vi "CD Read Engine.vi"(5 "Inline Status Channels Refs":T2[](array[typedef]) format="%.0x", 7 "Error (in)":errorcluster, 8 "RT Inline Data_Data Description_Channels":T3[](array[typedef]) {"Frame Drescriptors"."RT"."Status Channel Ref" format="%.0x"; "Frame Drescriptors"."RT"."Words Block Data Refs"."Data Reference" format="%.0x"; "Frame Drescriptors"."RT"."Timestamp Channel Data Reference" format="%.0x"; "Frame Drescriptors"."BC"."Status Channel Refs" format="%.0x"; "Frame Drescriptors"."BC"."Words Block Data Refs"."Data Reference" format="%.0x"; "Frame Drescriptors"."BC"."Timestamp Channel Data Reference" format="%.0x"}, 9 "Card Parameters (in)":T12) -> (0 "Error (out)":errorcluster, 3 "Array":T1[](array[typedef]) {"type" format="%04x"; "activity" format="%04x"; "error" format="%04x"; "cwd1" format="%04x"; "cwd2" format="%04x"; "swd1" format="%04x"; "swd2" format="%04x"; "data" format="%04x"})   [LabVIEW 2020, in "Ballard MIL-1553 Engine.lvlib"]
uses:
  Ballard MIL-1553 Engine.lvlib
  Controls/RT Inline Data_Data Description_Channel.ctl
  Controls/RT Inline Frame Descriptor.ctl
  Controls/RT Inline Frame Descriptor_BC.ctl
  <vilib>/NI VeriStand/Custom Device API/Data Reference.ctl
  <vilib>/NI VeriStand/Custom Device API/Block Data Reference.ctl
  <vilib>/NI VeriStand/Custom Device API/Custom Device Item Ref.ctl
  Controls/RT Inline Frame Descriptor_RT.ctl
  Shared/Controls and Global/RT CWD2.ctl
  Shared/Controls and Global/RT CWD1.ctl
  Shared/Controls and Global/RT messageType.ctl
  Controls/Card Parameters.ctl
  Shared/Controls and Global/Initialization Method.ctl
  <instrlib>/BTICardLib/Public/Controls/1553 Record.ctl
  <instrlib>/BTICardLib/BTICardLV.lvlib
  <vilib>/NI VeriStand/Custom Device Tools/Custom Device Utility Library/Custom Device Utility Library.lvlib
  Shared/Ballard 1553 Shared.lvlib
  <vilib>/NI VeriStand/Custom Device API/Custom Device API.lvlib
panel:
  in  "Tab Control":enum32{"Controls & Indicators", "Misc"}(tab)
  out "# of records read":i32
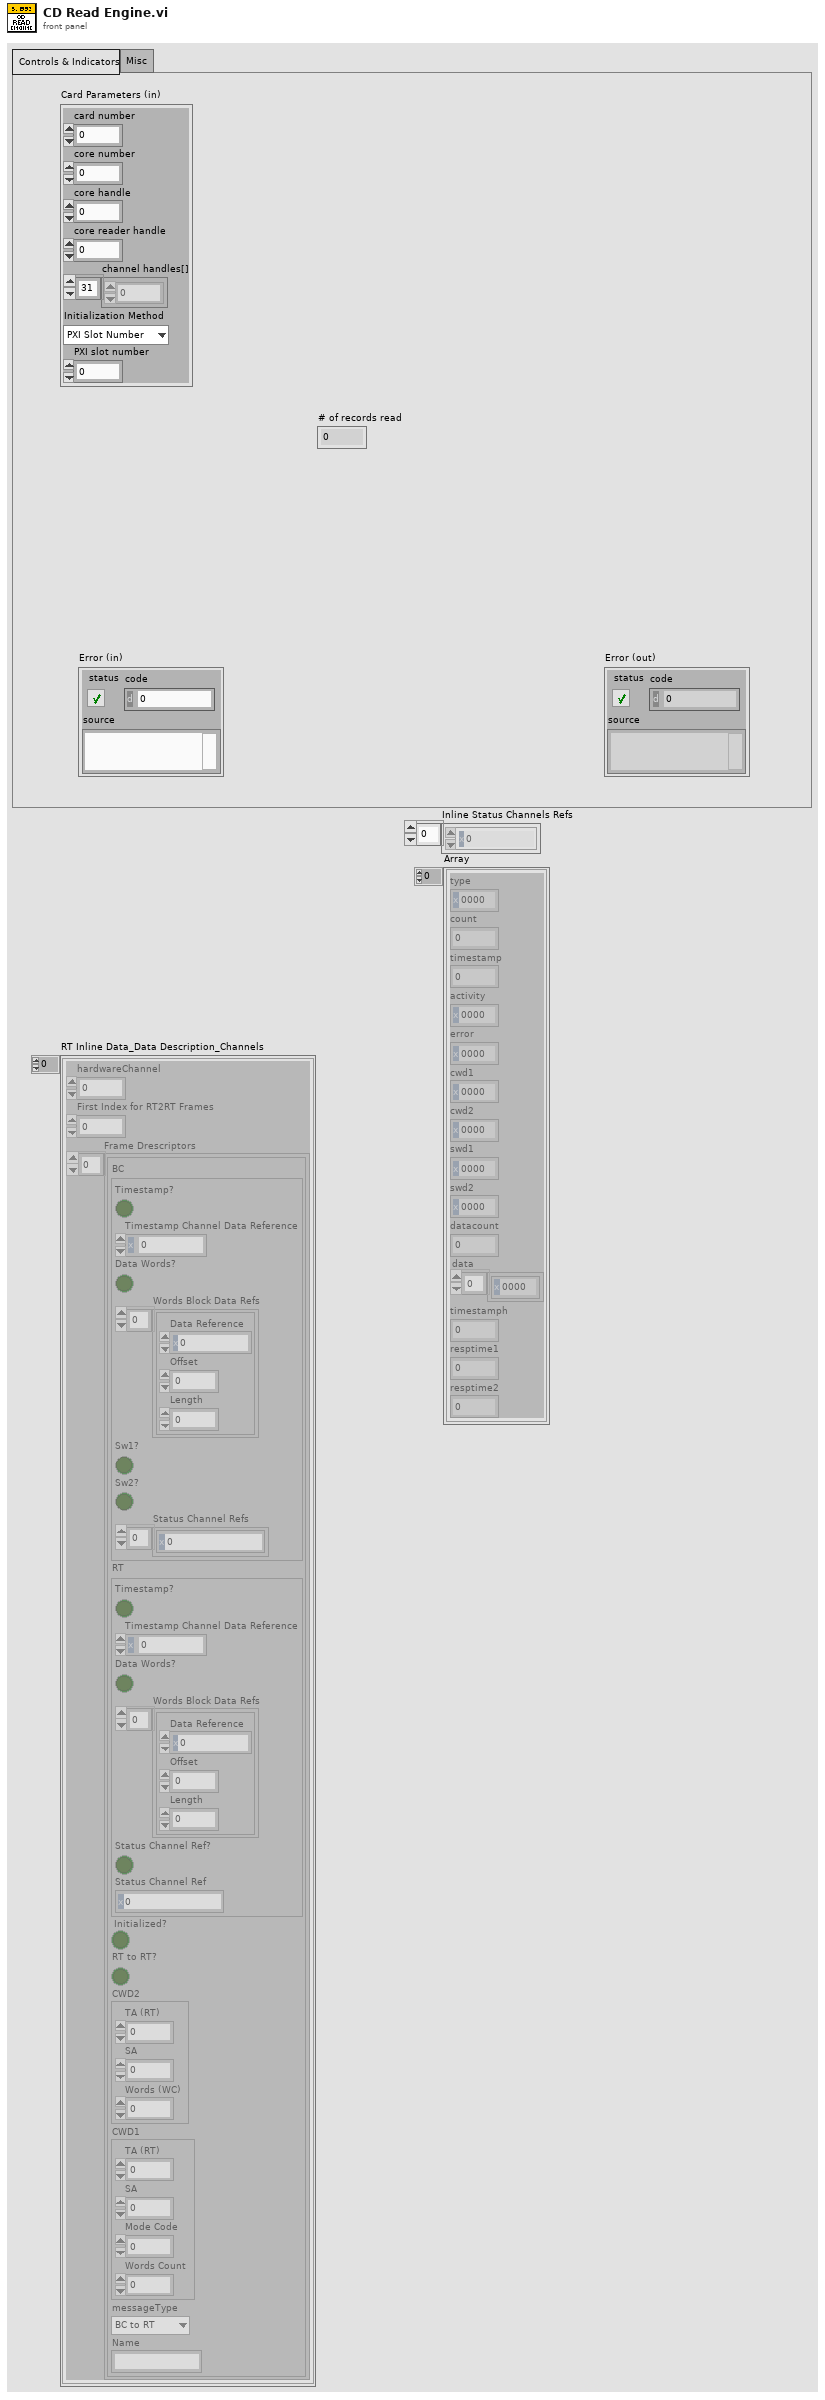
[diagram p1: front panel]
types:
  T1 = typedef "BTICardLV.lvlib/1553 Record.ctl" = cluster{"type":u16, "count":u16, "timestamp":u32, "activity":u16, "error":u16, "cwd1":u16, "cwd2":u16, "swd1":u16, "swd2":u16, "datacount":u16, "data":u16[], "timestamph":u32, "resptime1":u16, "resptime2":u16}
  T2 = typedef "Custom Device API.lvlib/Data Reference.ctl" = i32
  T3 = typedef "Ballard MIL-1553 Engine.lvlib/RT Inline Data_Data Description_Channel.ctl" = cluster{"hardwareChannel":u16, "First Index for RT2RT Frames":i32, "Frame Drescriptors":T4[]}
  T4 = typedef "Ballard MIL-1553 Engine.lvlib/RT Inline Frame Descriptor.ctl" = cluster{"BC":T5, "RT":T8, "Initialized?":bool, "RT to RT?":bool, "CWD2":T9, "CWD1":T10, "messageType":T11, "Name":string}
  T5 = typedef "Ballard MIL-1553 Engine.lvlib/RT Inline Frame Descriptor_BC.ctl" = cluster{"Timestamp?":bool, "Timestamp Channel Data Reference":T2, "Data Words?":bool, "Words Block Data Refs":T6[], "Sw1?":bool, "Sw2?":bool, "Status Channel Refs":T7[]}
  T6 = typedef "Custom Device API.lvlib/Block Data Reference.ctl" = cluster{"Data Reference":T2, "Offset":u64, "Length":u64}
  T7 = typedef "Custom Device API.lvlib/Custom Device Item Ref.ctl" = u64
  T8 = typedef "Ballard MIL-1553 Engine.lvlib/RT Inline Frame Descriptor_RT.ctl" = cluster{"Timestamp?":bool, "Timestamp Channel Data Reference":T2, "Data Words?":bool, "Words Block Data Refs":T6[], "Status Channel Ref?":bool, "Status Channel Ref":T7}
  T9 = typedef "Ballard 1553 Shared.lvlib/RT CWD2.ctl" = cluster{"TA (RT)":i8, "SA":i8, "Words (WC)":i8}
  T10 = typedef "Ballard 1553 Shared.lvlib/RT CWD1.ctl" = cluster{"TA (RT)":i8, "SA":i8, "Mode Code":i8, "Words Count":i8}
  T11 = typedef "Ballard 1553 Shared.lvlib/RT messageType.ctl" = enum16{"BC to RT", "RT to BC", "RT to RT", "MC (Rx)", "MC (Tx)"}
  T12 = typedef "Ballard MIL-1553 Engine.lvlib/Card Parameters.ctl" = cluster{"card number":i32, "core number":i32, "core handle":u64, "core reader handle":u64, "channel handles[]":u64[], "Initialization Method":T13, "PXI slot number":i32}
  T13 = typedef "Ballard 1553 Shared.lvlib/Initialization Method.ctl" = enum16{"PXI Slot Number", "Card Number"}
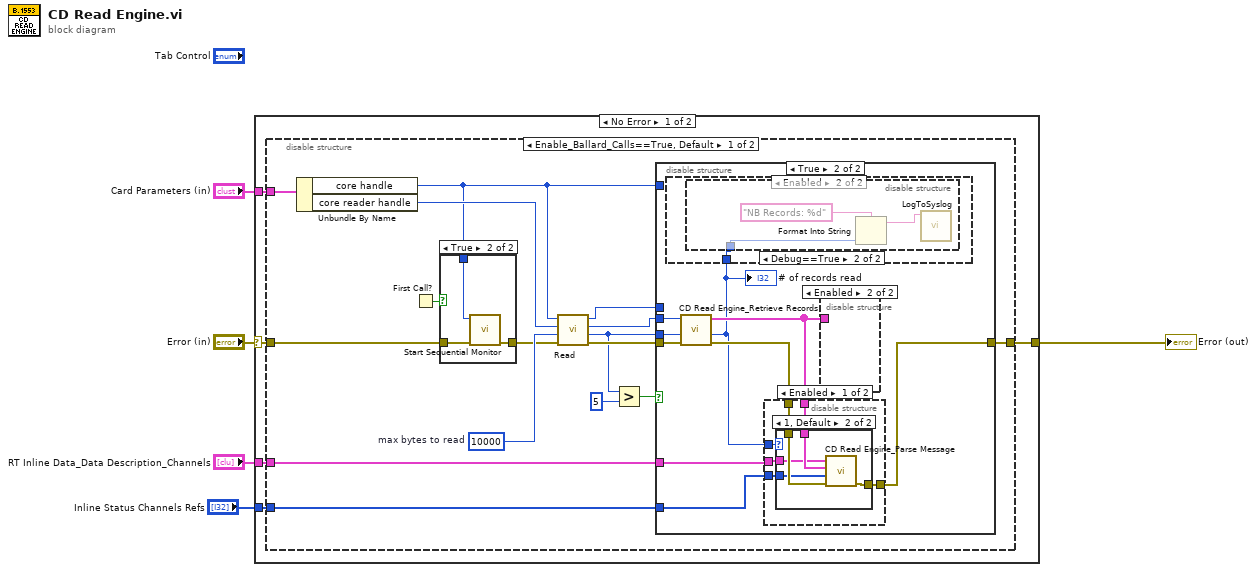
[diagram p0: block diagram]
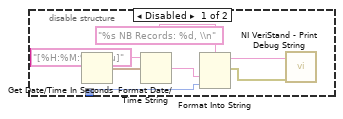
[diagram p3: hidden frame]
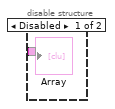
[diagram p5: hidden frame]
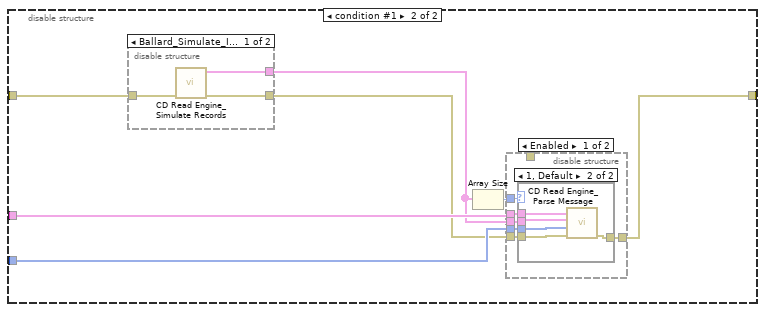
[diagram p9: hidden frame]
diagram:
  n1 = case shown="No Error" "Error (in)" {
    selector: "Error (in)" -> [w7 w90]
    tunnel: "Card Parameters (in)" -> [w10 _]
    tunnel: "RT Inline Data_Data Description_Channels" -> [w9 _]
    tunnel: [w8 w90] -> w3
    tunnel: "Inline Status Channels Refs" -> [w6 _]
    frame No Error {
      n2 = disable-structure shown="Enable_Ballard_Calls==True, Default" {
        disable-tunnel: w10 -> [w22 _]
        disable-tunnel: w9 -> [w21 w72]
        disable-tunnel: [w20 w71] -> w8
        disable-tunnel: w7 -> [w19 w69]
        disable-tunnel: w6 -> [w17 w70]
        frame condition #0 (active) {
          w25 = 10000  # max bytes to read
          n3 = Unbundle By Name(w22) -> ("core handle"=w11:u64, "core reader handle"=w26:u64)
          n4 = First Call?() -> (First Call?: T/F=w18:bool)
          n5 = case shown="True" w18 {
            tunnel: w11 -> [_ w65]
            tunnel: w19 -> [w62 w64]
            tunnel: [w62 w63] -> w16
            frame False {
            }
            frame True {
              n6 = call <instrlib>:"Start Sequential Monitor.vi"("error in (no error)"=w64, "core handle in"=w65) -> ("error out"=w63:errorcluster)  [unwired: 8 in, 1 out]
            }
          }
          n7 = call <instrlib>:"Read.vi"("error in (no error)"=w16, "max bytes to read"=w25, "core reader handle in"=w26, "core handle in"=w11) -> ("error out"=w23:errorcluster, "bytes read"=w13:i32, "core reader handle out"=w24:u64, "core handle out"=w12:u64)  [unwired: 4 in]
          n8 = Greater?(x=w13, y=5) -> (0:w15:bool)
          n9 = case shown="True" w15 {
            tunnel: w24 -> [_ w36]
            tunnel: w23 -> [w27 w35]
            tunnel: w21 -> [_ w34]
            tunnel: [w27 w33] -> w20
            tunnel: w17 -> [_ w32]
            tunnel: w13 -> [_ w29]
            tunnel: w12 -> [_ _]
            tunnel: w11 -> [_ _]
            frame False {
            }
            frame True {
              n10 = call "CD Read Engine_Retrieve Records.vi"("error in (no error)"=w35, "bytes read"=w29, "core reader handle in"=w36) -> ("error out"=w31:errorcluster, "# of records read"=w28:i32, "Array of Records"=w30:T1[])  [unwired: 6 in]
              "# of records read" <- w28
              n11 = disable-structure shown="Enabled" {
                disable-tunnel: w28 -> [w37 w44]
                frame Disabled {
                  n12 = Get Date/Time In Seconds() -> (seconds since 1Jan1904=w43:timestamp)
                  n13 = Format Date/Time String(time format string (%c)="[%H:%M:%S%3u]", seconds (now)=w43) -> (date/time string=w40:string)  [unwired: 1 in]
                  n14 = Format Into String(format string="%s NB Records: %d, \\n", w40, w37) -> (resulting string=w38:string, error out=w39:errorcluster)  [unwired: 2 in]
                  n15 = call <vilib>:"NI VeriStand - Print Debug String.vi"("error in (no error)"=w39, "Message"=w38) -> ()  [unwired: 9 in, 1 out]
                }
                frame Enabled {
                  n16 = disable-structure shown="Debug==True" {
                    disable-tunnel: w44 -> [_ w46]
                    frame condition #0 (active) {
                    }
                    frame condition #1 {
                      n17 = Format Into String(format string="NB Records: %d", w46) -> (resulting string=w45:string)  [unwired: 2 in, 1 out]
                      n18 = call "LogToSyslog.vi"("message"=w45) -> ()  [unwired: 9 in, 2 out]
                    }
                  }
                }
              }
              n19 = disable-structure shown="Enabled" {
                disable-tunnel: w34 -> [w50 _]
                disable-tunnel: [w54 w61] -> w33
                disable-tunnel: w31 -> [w53 w61]
                disable-tunnel: w32 -> [w52 _]
                disable-tunnel: w30 -> [w51 _]
                disable-tunnel: w28 -> [w49 _]
                frame Enabled {
                  n20 = case shown="1, Default" w49 {
                    tunnel: [w55 w60] -> w54
                    tunnel: w53 -> [w55 w59]
                    tunnel: w52 -> [_ w58]
                    tunnel: w51 -> [_ w57]
                    tunnel: w50 -> [_ w56]
                    frame 0 {
                    }
                    frame 1, Default {
                      n21 = call "CD Read Engine_Parse Message.vi"("Error (in)"=w59, "Inline Status Channels Refs"=w58, "Record []"=w57, "RT Inline Data_Data Description_Channels"=w56) -> ("Error (out)"=w60:errorcluster)  [unwired: 7 in]
                    }
                  }
                }
                frame Disabled {
                }
              }
              n22 = disable-structure shown="Enabled" {
                disable-tunnel: w30 -> [w48 _]
                frame Disabled {
                  "Array" <- w48
                }
                frame Enabled {
                }
              }
            }
          }
        }
        frame condition #1 {
          n23 = disable-structure shown="Ballard_Simulate_Inline==True" {
            disable-tunnel: w69 -> [w75 w76]
            disable-tunnel: [w74 w76] -> w68
            disable-tunnel: [w73 _] -> w67
            frame condition #0 {
              n24 = call "CD Read Engine_Simulate Records.vi"("error in (no error)"=w75) -> ("error out"=w74:errorcluster, "Record []"=w73:T1[])  [unwired: 9 in]
            }
            frame condition #1 (active) {
            }
          }
          n25 = Array Size(array=w67) -> (size(s)=w66:i32)
          n26 = disable-structure shown="Enabled" {
            disable-tunnel: w72 -> [w80 _]
            disable-tunnel: [w82 w89] -> w71
            disable-tunnel: _ -> [_ w89]
            disable-tunnel: w70 -> [w81 _]
            disable-tunnel: w68 -> [w79 _]
            disable-tunnel: w67 -> [w78 _]
            disable-tunnel: w66 -> [w77 _]
            frame Enabled {
              n27 = case shown="1, Default" w77 {
                tunnel: [w83 w88] -> w82
                tunnel: w81 -> [_ w87]
                tunnel: w80 -> [_ w86]
                tunnel: w79 -> [w83 w85]
                tunnel: w78 -> [_ w84]
                frame 0 {
                }
                frame 1, Default {
                  n28 = call "CD Read Engine_Parse Message.vi"("Error (in)"=w85, "Inline Status Channels Refs"=w87, "Record []"=w84, "RT Inline Data_Data Description_Channels"=w86) -> ("Error (out)"=w88:errorcluster)  [unwired: 7 in]
                }
              }
            }
            frame Disabled {
            }
          }
        }
      }
    }
    frame Error {
    }
  }
  "Error (out)" <- w3
